vi "Timer_Main_3.vi"() -> ()   [LabVIEW 2020]
uses:
  TimedDoor2_class/TimedDoor2.lvclass
  C:/Projects/DesignPatterns_Trunk/Timer/Door_class/Door.lvclass
panel:
  out "error out":errorcluster
  out "Sec":dbl
  out "Open?":bool
  in  "Close":bool
  in  "Open":bool
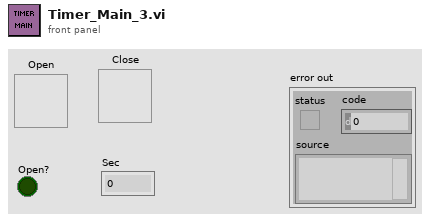
[diagram p1: front panel]
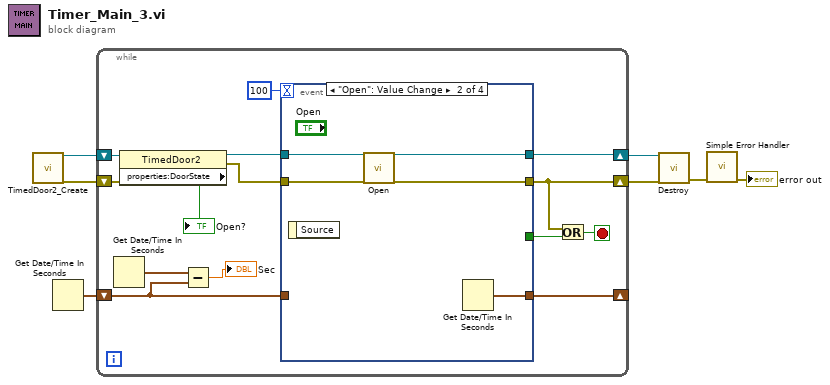
[diagram p0: block diagram]
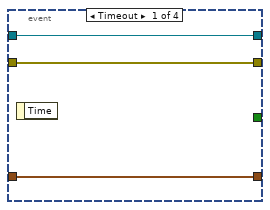
[diagram p2: hidden frame]
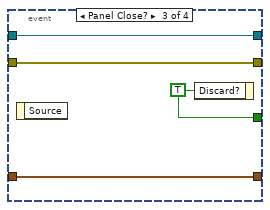
[diagram p3: hidden frame]
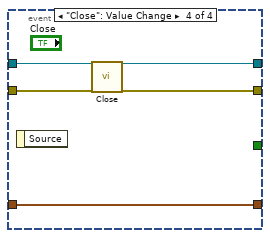
[diagram p4: hidden frame]
diagram:
  n1 = call "TimedDoor2_Create.vi"() -> ("reference out"=w7:refnum<class "TimedDoor2.lvclass">, "error out"=w6:errorcluster)  [unwired: 18 in]
  n2 = Get Date/Time In Seconds() -> (seconds since 1Jan1904=w2:timestamp)
  n3 = while {
    shift-right: [w17] -> w5
    shift-left: w7 -> [w20]
    shift-right: [w14] -> w4
    shift-left: w6 -> [w19]
    shift-right: [w11] -> _
    shift-left: w2 -> [w8]
    stop <- w12 stop-if-true
    n4 = Get Date/Time In Seconds() -> (seconds since 1Jan1904=w10:timestamp)
    n5 = property class="TimedDoor2"(reference=w20, error in=w19) -> (reference out=w18:refnum<class "TimedDoor2.lvclass">, error out=w16:errorcluster, "properties:DoorState"=→"Open?":bool)
    n6 = Subtract(x=w10, y=w8) -> (x-y=→"Sec":dbl)
    n7 = event shown="[1] \"Open\": Value Change" {
      selector: _ -> [_ _ _ _]
      dyn-events: _ -> [_ _ _ _]
      timeout: 100 -> [_ _ _ _]
      tunnel: w18 -> [w24 w29 w32 w38]
      tunnel: [w24 w26 w32 w35] -> w17
      tunnel: w16 -> [w23 w28 w33 w37]
      tunnel: [w23 w27 w33 w36] -> w14
      tunnel: [_ _ w31 _] -> w13
      tunnel: [w22 w25 w30 w34] -> w11
      tunnel: w8 -> [w22 _ w30 w34]
      event Timeout {
        n8 = event-data() -> ()  [unwired: 1 in, 1 out]
      }
      event "Open": Value Change {
        n9 = event-data() -> ()  [unwired: 1 in, 1 out]
        n10 = call-dynamic "Open.vi"("reference in"=w29, "Error In"=w28) -> ("reference in"=w26:refnum<class "TimedDoor2.lvclass">, "Error Out"=w27:errorcluster)  [unwired: 16 in]
        n11 = Get Date/Time In Seconds() -> (seconds since 1Jan1904=w25:timestamp)
      }
      event Panel Close? {
        w31 = TRUE ("Discard?")
        n12 = event-data() -> ()  [unwired: 1 in, 1 out]
        n13 = event-data("Discard?"=w31) -> ()  [unwired: 1 in, 1 out]
      }
      event "Close": Value Change {
        n14 = event-data() -> ()  [unwired: 1 in, 1 out]
        n15 = call-dynamic "Close.vi"("reference in"=w38, "error in (no error)"=w37) -> ("reference out"=w35:refnum<class "TimedDoor2.lvclass">, "error out"=w36:errorcluster)  [unwired: 16 in]
      }
    }
    n16 = Or(x=w14, y=w13) -> (x .or. y?=w12:bool)
  }
  n17 = call-dynamic "Destroy.vi"("reference in"=w5, "error in (no error)"=w4) -> ("error out"=w3:errorcluster)  [unwired: 16 in, 1 out]
  n18 = call <vilib>:"Simple Error Handler.vi"("error in (no error)"=w3) -> ("error out"=→"error out":errorcluster)  [unwired: 4 in, 4 out]
